vi "Stop Core.vi"(10 "final error code":i32, 11 "DLS Laser Actor in":refnum<class "FLS Laser Actor.lvclass">) -> (3 "DLS Laser Actor out":refnum<class "FLS Laser Actor.lvclass">)   [LabVIEW 2018, in "FLS Laser Actor.lvlib" / "FLS Laser Actor.lvclass"]
doc: "In addition to the following, this method also sends a message to the monitor to notify it that the actor has stopped execution.\n\n(<B>Filename</B>: Actor Framework.lvlib:Actor.lvclass:Stop Core.vi)\n\nDefines what the actor does before it stops. Use the <B>final error code</B> input to determine whether the actor shut down in response to an error.\n\nBy default, this method does nothing. A descendant class may override it to define behavior, such as shutting down any processes the actor initiated in its override of the Actor Core method.\n\nCopyright: MGI\nAuthored by: Derek Trepanier"
uses:
  FLS Laser Actor.lvclass
  FLS Laser Actor.lvclass/FLS Laser Actor.ctl
  Actor Monitor/Actor/Monitored Actor.lvclass
panel:
  out "error out":errorcluster
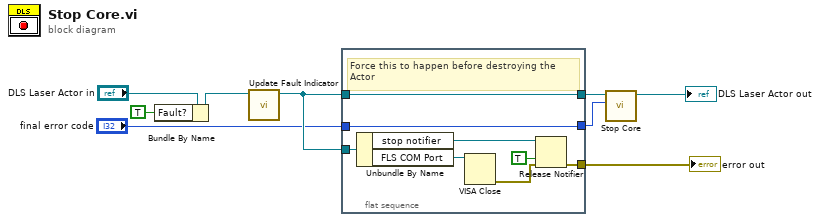
[diagram p0: block diagram]
diagram:
  n1 = Bundle By Name(cluster="DLS Laser Actor in", "Fault?"=TRUE) -> (w5:refnum<class "FLS Laser Actor.lvclass">)
  n2 = call "Update Fault Indicator.vi"("DLS Laser Actor in"=w5) -> ("DLS Laser Actor out"=w4:refnum<class "FLS Laser Actor.lvclass">)  [unwired: 9 in, 1 out]
  n3 = flat-sequence {
    tunnel: [w13] -> w8
    tunnel: w4 -> [w12]
    tunnel: w4 -> [w11]
    tunnel: [w11] -> w3
    tunnel: "final error code" -> [w10]
    tunnel: [w10] -> w1
    frame #0 {
      # "Force this to happen before destroying the Actor"
      n4 = Unbundle By Name(w12) -> ("stop notifier"=w17:refnum<notifier>, "FLS COM Port"=w15:refnum<visa-resource-name>)
      n5 = VISA Close(VISA resource name=w15) -> (error out=w14:errorcluster)  [unwired: 1 in]
      n6 = Release Notifier(notifier=w17, force destroy? (F)=TRUE, error in (no error)=w14) -> (error out=w13:errorcluster)  [unwired: 2 out]
    }
  }
  n7 = call-parent "Stop Core.vi"("final error code"=w1, "Monitored Actor in"=w3) -> ("Monitored Actor out"=→"DLS Laser Actor out":refnum<class "FLS Laser Actor.lvclass">)  [unwired: 9 in]
  "error out" <- w8
